vi "Dashboard Vision Processing.vi"(9 "LED Color":T5={"Hue"={35.0, 169.0}, "Sat"={140.0, 255.0}, "Val"={146.0, 255.0}} {"Hue" scale=0.0..255.0 scale format="%#_3g"}, 11 "Camera Image":T1) -> (1 "Detected Targets":T2(array[cluster]) {"Normalized Rect"."Numeric 5" format="%#_2g"; "Normalized Rect"."Numeric 3" format="%#_2g"; "Normalized Rect"."Numeric 2" format="%#_2g"; "Normalized Rect"."Numeric" format="%#_2g"}, 3 "Orig Image":T1(plugin-control))   [LabVIEW 2015]
uses:
  Vision Support Code/Camera Types.ctl
  <vilib>/vision/Image Controls.llb/IMAQ Image.ctl
  <vilib>/vision/NI_Vision_Development_Module.lvlib
panel:
  out "Highest Avg Score":dbl
  out "Sorted Particle Scores":T3(array[cluster]) {"Moment Factor" format="%#_3g"; "Aspect Ratio" format="%#_3g"; "Area to CH" format="%#_3g"; "X" format="%#_3g"; "Y" format="%#_3g"}
  in  "Display Original":bool=TRUE
  out "Original Image":T1(plugin-control)
  in  "Emphasize Limit Tests":bool=TRUE
  in  "Camera Type":T4=enum."MS HD3000 square"
  in  "Min Score Threshold":i32=75
  in  "Aspect Fudge Factor":dbl=1.0
  in  "Score Threshold":dbl=75.0
  out "Qualified Particles":i32
  # "Density Profile"
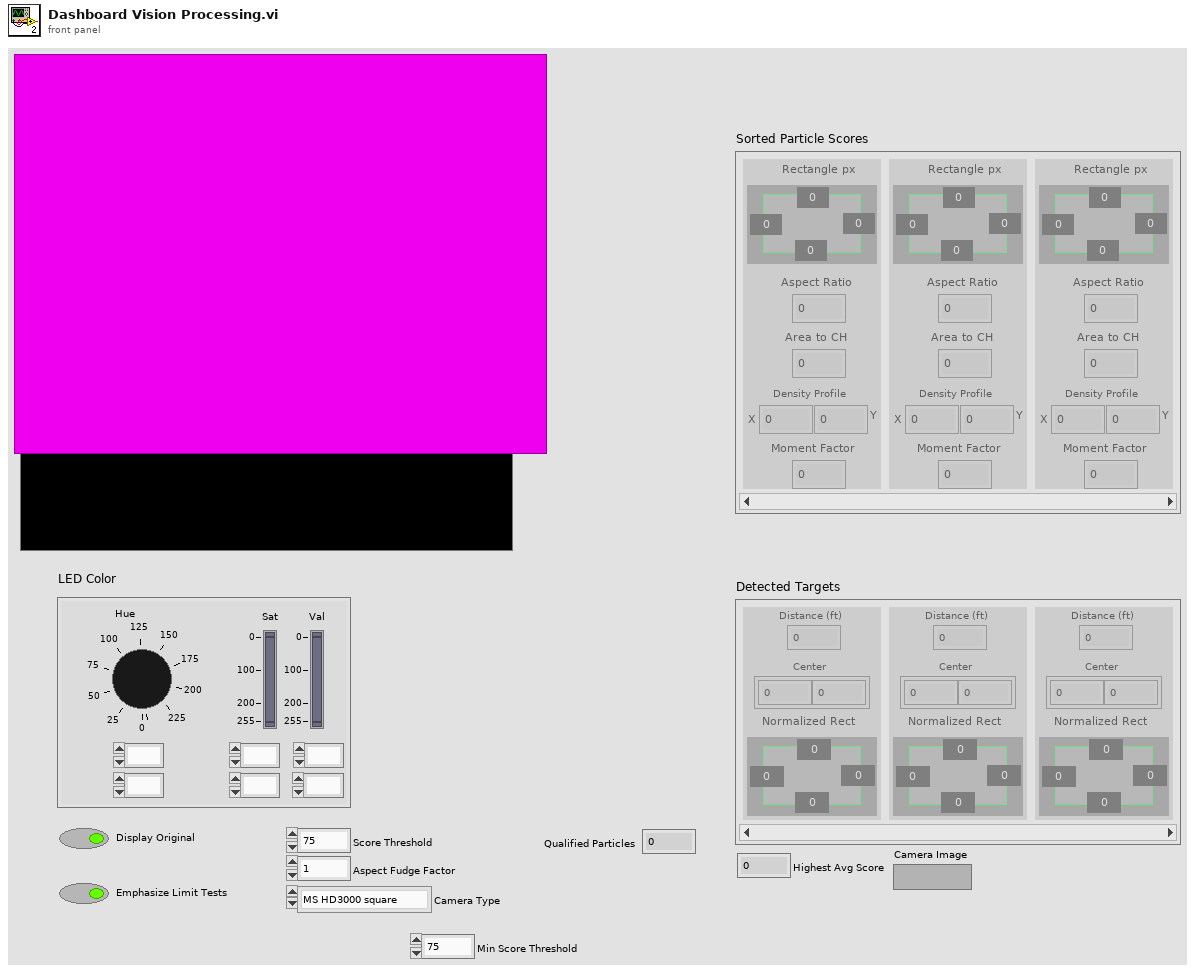
[diagram p1: front panel]
types:
  T1 = typedef "IMAQ Image.ctl" = refnum<image>
  T2 = cluster{"Distance (ft)":dbl, "Center":cluster{dbl, dbl}, "Normalized Rect":cluster{"Numeric":dbl, "Numeric 2":dbl, "Numeric 3":dbl, "Numeric 5":dbl}}[]
  T3 = cluster{"Rectangle px":cluster{"Numeric":dbl, "Numeric 2":dbl, "Numeric 3":dbl, "Numeric 5":dbl}, "Aspect Ratio":dbl, "Area to CH":dbl, "X":dbl, "Y":dbl, "Moment Factor":dbl}[]
  T4 = typedef "Camera Types.ctl" = enum16{"206", "1011", "1013", "MS HD3000 square", "MS HD3000 640x480"}
  T5 = cluster{"Hue":cluster{dbl, dbl}, "Sat":cluster{dbl, dbl}, "Val":cluster{dbl, dbl}}
  T6 = typedef "Image Type" = u32
  T7 = typedef "Particle Parameters" = i32
  T8 = cluster{"Bounding box":cluster{"left":dbl, "top":dbl, "right":dbl, "bottom":dbl}, "Aspect Ratio":dbl, "Area to CH":dbl, "X Mask":dbl, "Y Mask":dbl, "Moment":dbl}[]
  T9 = cluster{"Rectangle":cluster{"Numeric":dbl, "Numeric 2":dbl, "Numeric 3":dbl, "Numeric 5":dbl}, "L":dbl, "Area to CH":dbl, "X":dbl, "Y":dbl, "Moment Factor":dbl}[]
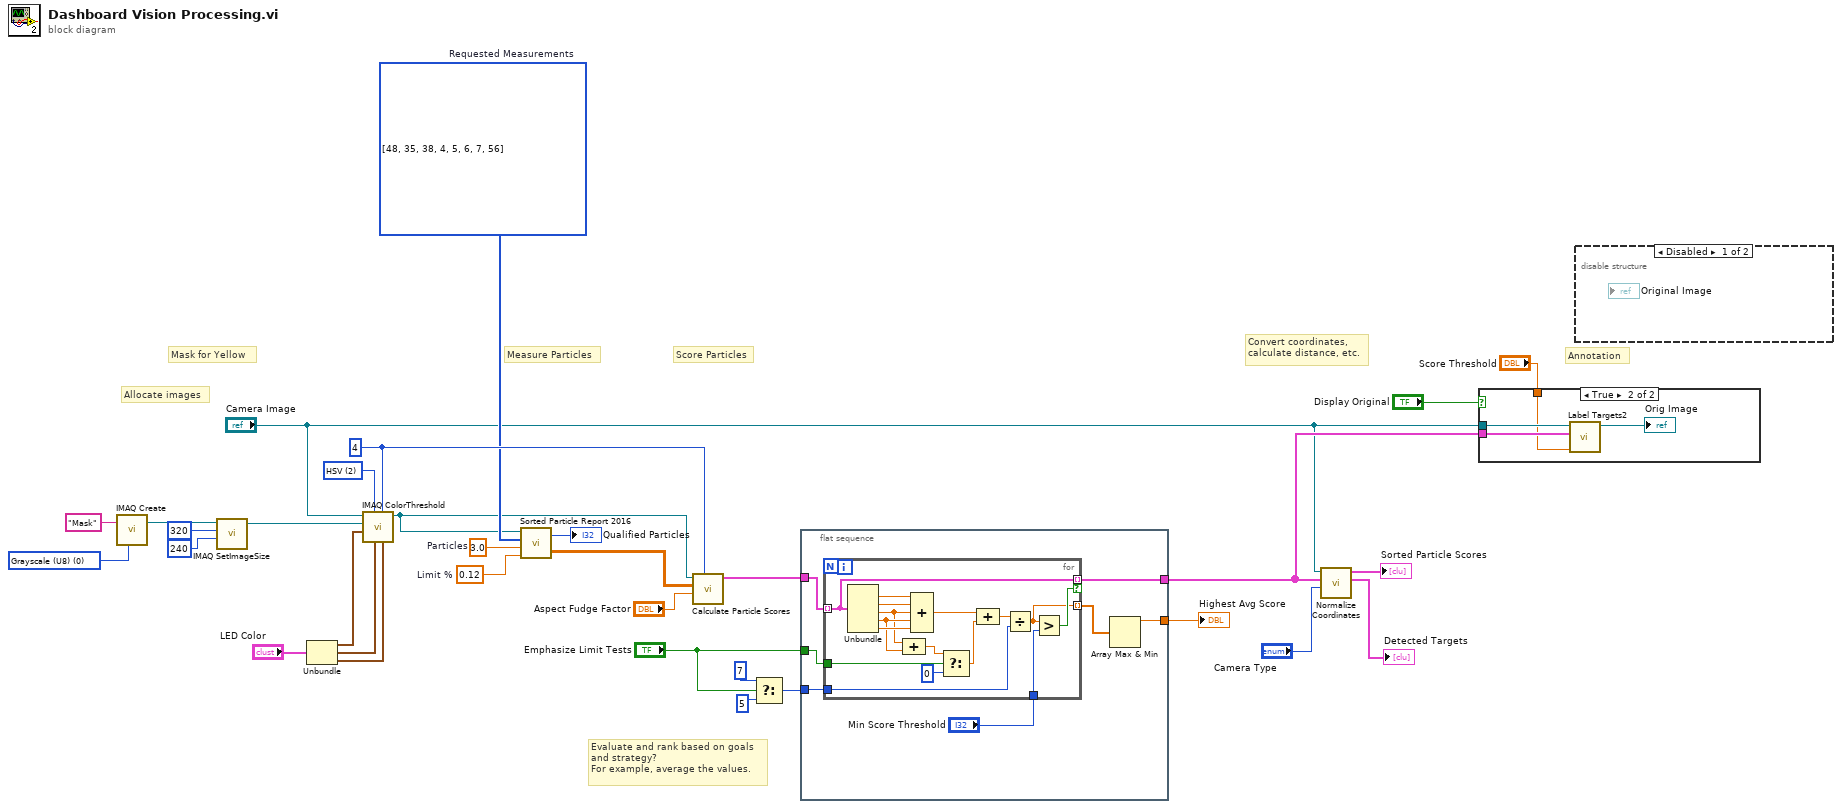
[diagram p0: block diagram]
diagram:
  w8 = T6 0 items=["Grayscale (U8)", "Grayscale (I16)", "Grayscale (SGL)", "Complex (CSG)", "RGB (U32)", "HSL (U32)", "RGB (U64)", "Grayscale (U16)"] ("Image Type")
  w13 = T7[] [48, 35, 38, 4, 5, 6, 7, 56] items=["Center of Mass X", "Center of Mass Y", "First Pixel X", "First Pixel Y", "Bounding Rect Left", "Bounding Rect Top", "Bounding Rect Right", "Bounding Rect Bottom", "Max Feret Diameter Start X", "Max Feret Diameter Start Y", "Max Feret Diameter End X", "Max Feret Diameter End Y", "Max Horiz. Segment Length Left", "Max Horiz. Segment Length Right", "Max Horiz. Segment Length Row", "-", "Bounding Rect Width", "Bounding Rect Height", "Bounding Rect Diagonal", "Perimeter", "Convex Hull Perimeter", "Holes' Perimeter", "Max Feret Diameter", "Equivalent Ellipse Major Axis", "Equivalent Ellipse Minor Axis", "Equivalent Ellipse Minor Axis (Feret)", "Equivalent Rect Long Side", "Equivalent Rect Short Side", "Equivalent Rect Diagonal", "Equivalent Rect Short Side (Feret)", "Average Horiz. Segment Length", "Average Vert. Segment Length", "Hydraulic Radius", "Waddel Disk Diameter", "-", "Area", "Holes' Area", "Particle & Holes' Area", "Convex Hull Area", "Image Area", "-", "Number of Holes", "Number of Horiz. Segments", "Number of Vert. Segments", "-", "Orientation", "Max Feret Diameter Orientation", "-", "% Area/Image Area", "% Area/(Particle & Holes' Area)", "Ratio of Equivalent Ellipse Axes", "Ratio of Equivalent Rect Sides", "-", "Elongation Factor", "Compactness Factor", "Heywood Circularity Factor", "Type Factor", "-", "Sum X", "Sum Y", "Sum XX", "Sum XY", "Sum YY", "Sum XXX", "Sum XXY", "Sum XYY", "Sum YYY", "-", "Moment of Inertia XX", "Moment of Inertia XY", "Moment of Inertia YY", "Moment of Inertia XXX", "Moment of Inertia XXY", "Moment of Inertia XYY", "Moment of Inertia YYY", "Norm. Moment of Inertia XX", "Norm. Moment of Inertia XY", "Norm. Moment of Inertia YY", "Norm. Moment of Inertia XXX", "Norm. Moment of Inertia XXY", "Norm. Moment of Inertia XYY", "Norm. Moment of Inertia YYY", "Hu Moment 1", "Hu Moment 2", "Hu Moment 3", "Hu Moment 4", "Hu Moment 5", "Hu Moment 6", "Hu Moment 7"]  # Requested Measurements
  w16 = 4 ("Replace Value")
  w28 = u16 2 items=["RGB", "HSL", "HSV", "HSI"] ("Color Mode")
  w30 = 0.12  # Limit %
  w32 = 3.0  # Particles
  # "Allocate images"
  # "Evaluate and rank based on goals\nand strategy?\nFor example, average the values."
  # "Measure Particles"
  # "Convert coordinates,\ncalculate distance, etc."
  # "Annotation"
  # "Score Particles"
  # "Mask for Yellow"
  n1 = call "IMAQ Create"("Image Name"="Mask", "Image Type"=w8) -> ("New Image"=w4:T1)  [unwired: 2 in, 2 out]
  n2 = call "IMAQ SetImageSize"("Y Resolution"=240, "X Resolution"=320, "Image"=w4) -> ("Image Out"=w3:T1)  [unwired: 2 in, 1 out]
  n3 = Unbundle("LED Color") -> ("Hue"=w12:cluster{dbl, dbl}, "Sat"=w11:cluster{dbl, dbl}, "Val"=w10:cluster{dbl, dbl})
  n4 = call "IMAQ ColorThreshold"("Blue or Luma or Val or Inten Range"=w10, "Replace Value"=w16, "Green or Sat Range"=w11, "Color Mode"=w28, "Red or Hue Range"=w12, "Image Dst"=w3, "Image Src"="Camera Image") -> ("Image Dst Out"=w5:T1)  [unwired: 3 in, 1 out]
  n5 = call "Sorted Particle Report 2016.vi"("Min Area Size %"=w30, "Particle Count Limit"=w32, "Pixel Measurements"=w13, "Image in"=w5) -> ("Sorted Data"=w27:dbl[][], "Particles"=→"Qualified Particles":i32)
  n6 = call "Calculate Particle Scores.vi"("Pixel Value"=w16, "Aspect Fudge Factor"="Aspect Fudge Factor", "Sorted Data"=w27, "Image in"=w5) -> ("Scores"=w25:T8)  [unwired: 7 in]
  n7 = Select(t=7, s="Emphasize Limit Tests", f=5) -> (s? t:f=w22:i32)
  n8 = flat-sequence {
    tunnel: w25 -> [w38]
    tunnel: w22 -> [w36]
    tunnel: [w39] -> w21
    tunnel: [w33] -> w18
    tunnel: "Emphasize Limit Tests" -> [w37]
    frame #0 {
      n9 = for {
        tunnel: w38 -> [w53] mode=indexing
        tunnel: [w53] -> w33 mode=indexing if=w52
        tunnel: [w51] -> w34 mode=indexing
        tunnel: w36 -> [w50]
        tunnel: "Min Score Threshold" -> [w49]
        tunnel: w37 -> [w42]
        n10 = Unbundle(w53) -> ("Aspect Ratio"=w55:dbl, "Area to CH"=w54:dbl, "X Mask"=w44:dbl, "Y Mask"=w45:dbl, "Moment"=w46:dbl)  [unwired: 1 out]
        n11 = Compound Arithmetic op=ADD(w44, w45) -> (w43:dbl)
        n12 = Compound Arithmetic op=ADD(w55, w54, w44, w45, w46) -> (w48:dbl)
        n13 = Select(t=w43, s=w42, f=0) -> (s? t:f=w41:dbl)
        n14 = Compound Arithmetic op=ADD(w48, w41) -> (w47:dbl)
        n15 = Divide(x=w47, y=w50) -> (x/y=w51:dbl)
        n16 = Greater?(x=w51, y=w49) -> (0:w52:bool)
      }
      n17 = Array Max & Min(array=w34) -> (max value=w39:dbl)  [unwired: 3 out]
    }
  }
  n18 = call "Normalize Coordinates.vi"("Camera Type"="Camera Type", "Targets"=w18, "Image in"="Camera Image") -> ("Found Targets"=→"Detected Targets":T2, "Sorted Scores"=→"Sorted Particle Scores":T9)  [unwired: 7 in]
  n19 = case shown="True" "Display Original" {
    tunnel: "Camera Image" -> [_ w59]
    tunnel: w18 -> [_ w58]
    tunnel: "Score Threshold" -> [_ w57]
    frame False {
    }
    frame True {
      n20 = call "Label Targets2.vi"("Score Threshold"=w57, "Targets"=w58, "Image in"=w59) -> ("Image out"=→"Orig Image":T1)  [unwired: 8 in]
    }
  }
  n21 = disable-structure shown="Disabled" {
    frame Disabled {
    }
    frame Enabled {
    }
  }
  "Highest Avg Score" <- w21
